vi "Register and Use Kernel Events.vi"() -> ()   [LabVIEW 2012]
uses:
  User Controls/Array Dimensions.ctl
  Non-User VIs/Allocate Memory/AllocateMemory_32f.vi
  Non-User VIs/Set Kernel Arguments/Set Kernel Arguments Memory Object.vi
  Non-User VIs/Error Checking/View Error Log Mode Functional Global.vi
  Non-User VIs/Read Memory/ReadMemory_32f.vi
  OpenCLV x64.lvlib
panel:
  out "Intensity Graph":sgl[][](graph)
  in  "Stop Button":bool
  in  "Slider":dbl(slide) scale=0.0..10.0
  in  "Gauge":dbl(knob) scale=0.0..10.0
  in  "Test Events":bool
  # "Press Test Events and still have control over the UI"
  # "Note:  If running on the CPU, the processer usage will hit 100%, but there is still UI control\nTry running on a GPU as well, though it may finish very quickly!"
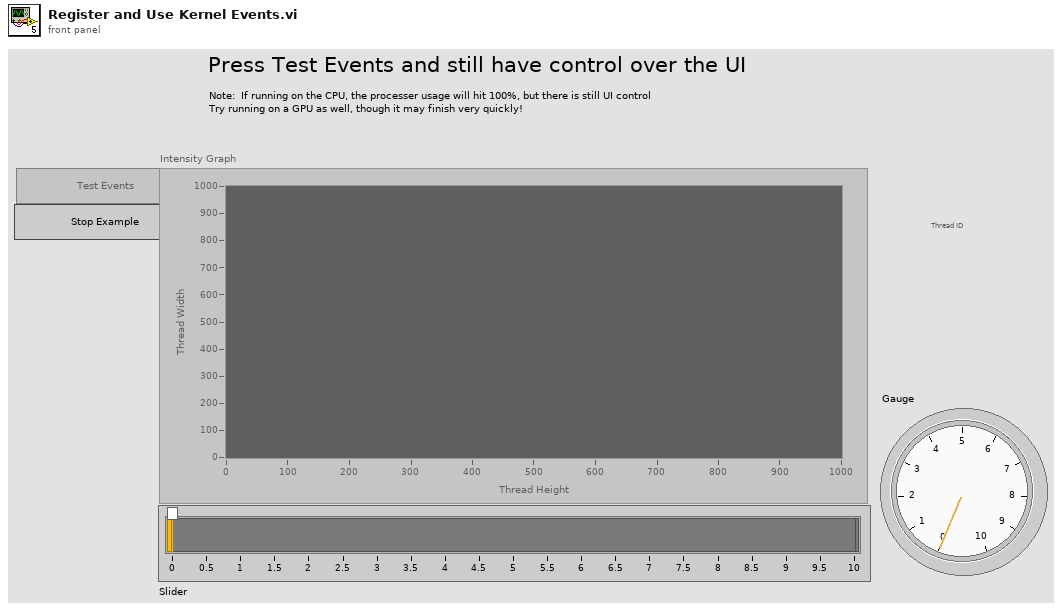
[diagram p1: front panel]
types:
  T1 = enum8{"Enabled", "Disabled", "Disabled and Grayed Out"}
  T2 = typedef "Array Dimensions.ctl" = cluster{"Depth":u64, "Height":u64, "Width":u64}
  T3 = typedef "OpenCLV x64.lvlib/Device ID.ctl" = u64
  T4 = typedef "OpenCLV x64.lvlib/Memory Object.ctl" = cluster{"Device ID":T3, "Memeroy ID":T5, "Dimension":T2, "Memory Type":T6}
  T5 = typedef "OpenCLV x64.lvlib/Memory ID.ctl" = u64
  T6 = typedef "OpenCLV x64.lvlib/Memory Type.ctl" = enum16{"32f", "u8", "i8", "u16", "i16", "u32", "i32", "64f"}
  T7 = typedef "OpenCLV x64.lvlib/Program Handle.ctl" = u64
  T8 = typedef "OpenCLV x64.lvlib/Kernel Handle.ctl" = u64
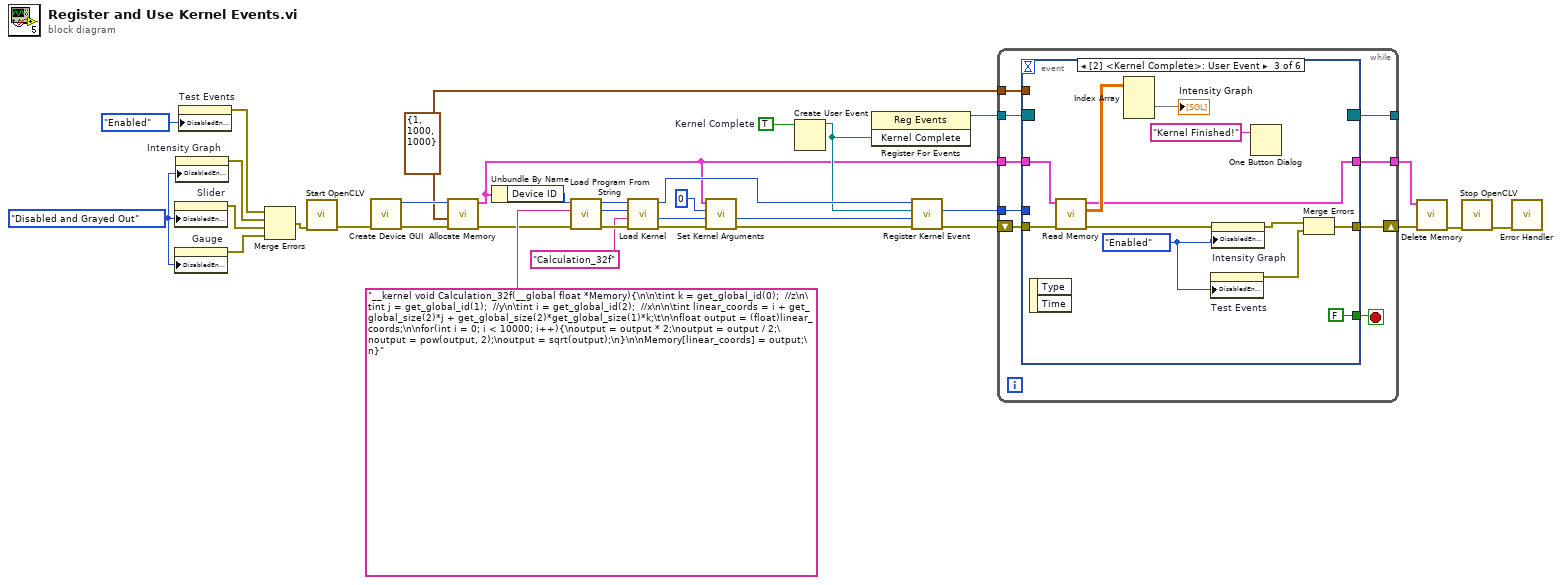
[diagram p0: block diagram]
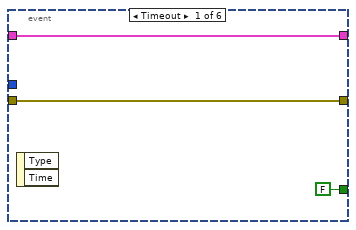
[diagram p2: hidden frame]
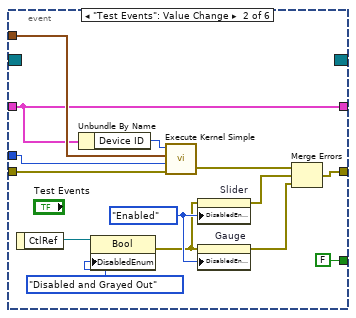
[diagram p3: hidden frame]
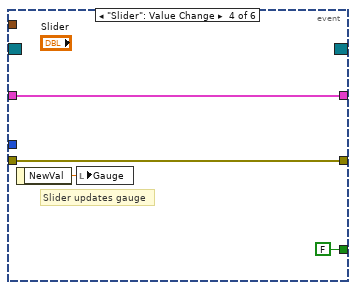
[diagram p4: hidden frame]
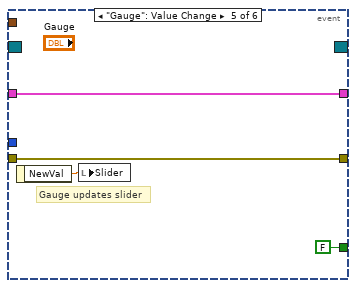
[diagram p5: hidden frame]
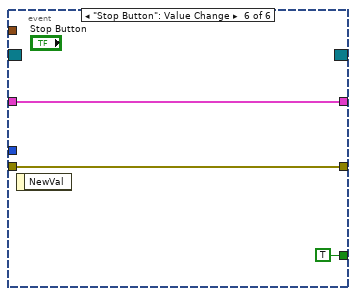
[diagram p6: hidden frame]
diagram:
  w13 = T1."Disabled and Grayed Out" ("Disabled")
  w24 = T2 {"Depth"=1, "Height"=1000, "Width"=1000} ("Dimension")
  w28 = TRUE  # Kernel Complete
  n1 = property on="Slider" class="Slide (strict)"("DisabledEnum"=w13) -> (error out=w17:errorcluster)  [unwired: 2 in, 1 out]
  n2 = property on="Gauge" class="Knob (strict)"("DisabledEnum"=w13) -> (error out=w16:errorcluster)  [unwired: 2 in, 1 out]
  n3 = property on="Intensity Graph" class="IntGraph (strict)"("DisabledEnum"=w13) -> (error out=w12:errorcluster)  [unwired: 2 in, 1 out]
  n4 = property on="Test Events" class="Bool"("DisabledEnum"=T1."Enabled" ("Disabled")) -> (error out=w10:errorcluster)  [unwired: 2 in, 1 out]
  n5 = Merge Errors(w10, w12, w17, w16) -> (w18:errorcluster)
  n6 = call "Start OpenCLV.vi"("Error In"=w18) -> ("Error Out"=w34:errorcluster)  [unwired: 10 in]
  n7 = call "Create Device GUI.vi"("Error In"=w34) -> ("error constant"=w26:errorcluster, "Device Reference"=w25:T3)  [unwired: 9 in]
  n8 = call-poly "Allocate Memory.vi"("Error In"=w26, "Dimension"=w24, "Device In"=w25) -> ("Error Out"=w23:errorcluster, "Memory Object"=w3:T4)  [unwired: 6 in, 1 out]
  n9 = Unbundle By Name(w3) -> ("Device ID"=w19:T3)
  n10 = call "Load Program From String.vi"("Error In"=w23, "OpenCL Source Code"="__kernel void Calculation_32f(__global float *Memory){\n\n\tint k = get_global_id(0);  //z\n\tint j = get_global_id(1);  //y\n\tint i = get_global_id(2);  //x\n\n\tint linear_coords = i + get_global_size(2)*j + get_global_size(2)*get_global_size(1)*k;\t\n\nfloat output = (float)linear_coords;\n\nfor(int i = 0; i < 10000; i++){\noutput = output * 2;\noutput = output / 2;\noutput = pow(output, 2);\noutput = sqrt(output);\n}\n\nMemory[linear_coords] = output;\n}", "Device In"=w19) -> ("Error Out"=w31:errorcluster, "Program Handle"=w30:T7, "Device Out"=w32:T3)  [unwired: 6 in]
  n11 = call "Load Kernel.vi"("Error In"=w31, "Kernel Name"="Calculation_32f", "Program Handle"=w30, "Device In"=w32) -> ("Error Out"=w22:errorcluster, "Kernel Handle"=w21:T8, "Device Out"=w6:T3)  [unwired: 4 in, 1 out]
  n12 = call-poly "Set Kernel Arguments.vi"("Error In"=w22, "Kernel Handle"=w21, "Argument Number"=0, "Memory Object"=w3) -> ("Error Out"=w8:errorcluster, "Kernel Handle out"=w7:T8)  [unwired: 5 in, 1 out]
  n13 = Create User Event(user event datatype=w28) -> (user event=w5:refnum<user-event>)  [unwired: 1 in, 1 out]
  n14 = register-events(w5) -> (reference out=w27:refnum<event-registration>)  [unwired: 2 in, 1 out]
  n15 = call "Register Kernel Event.vi"("Error In"=w8, "Kernel Handle"=w7, "User Event"=w5, "Device ID"=w6) -> ("Error Out"=w9:errorcluster, "Kernel Handle Out"=w1:T8)  [unwired: 4 in, 2 out]
  n16 = while {
    tunnel: w27 -> [w43]
    tunnel: w24 -> [w40]
    shift-right: [w39] -> w14
    shift-left: w9 -> [w42]
    tunnel: [w38] -> _
    tunnel: w3 -> [w37]
    tunnel: [w36] -> w4
    tunnel: w1 -> [w35]
    stop <- w41 stop-if-true
    n17 = event shown="[2] <Kernel Complete>: User Event" {
      selector: w43 -> [_ _ _ _ _ _]
      dyn-events: [_ _ _ _ _ _] -> w38
      timeout: _ -> [_ _ _ _ _ _]
      tunnel: w42 -> [w45 w60 w71 w74 w78 w83]
      tunnel: [FALSE FALSE FALSE FALSE FALSE TRUE] -> w41
      tunnel: w40 -> [_ w59 _ _ _ _]
      tunnel: [w45 w54 w69 w74 w78 w83] -> w39
      tunnel: w37 -> [w44 w48 w62 w73 w77 w81]
      tunnel: [w44 w48 w61 w73 w77 w81] -> w36
      tunnel: w35 -> [_ w47 _ _ _ _]
      event Timeout {
        n18 = event-data() -> ()  [unwired: 1 in, 2 out]
      }
      event "Test Events": Value Change {
        w58 = T1."Enabled" ("Disabled")
        n19 = event-data() -> ("CtlRef"=w57:refnum<vi>)  [unwired: 1 in]
        n20 = Unbundle By Name(w48) -> ("Device ID"=w49:T3)
        n21 = property class="Bool"(reference=w57, "DisabledEnum"=T1."Disabled and Grayed Out" ("Disabled")) -> (error out=w55:errorcluster)  [unwired: 1 in, 1 out]
        n22 = call "Execute Kernel Simple.vi"("Error In"=w60, "Kernel Handle"=w47, "Thread Dimensions"=w59, "Device In"=w49) -> ("Error Out"=w51:errorcluster)  [unwired: 4 in, 3 out]
        n23 = property on="Slider" class="Slide (strict)"(error in=w55, "DisabledEnum"=w58) -> (error out=w52:errorcluster)  [unwired: 1 in, 1 out]
        n24 = property on="Gauge" class="Knob (strict)"(error in=w55, "DisabledEnum"=w58) -> (error out=w53:errorcluster)  [unwired: 1 in, 1 out]
        n25 = Merge Errors(w51, w52, w53) -> (w54:errorcluster)
      }
      event User Event {
        w63 = T1."Enabled" ("Disabled")
        n26 = event-data() -> ()  [unwired: 1 in, 2 out]
        n27 = call-poly "Read Memory.vi"("Error In"=w71, "Memory Object In"=w62) -> ("Error Out"=w65:errorcluster, "Data Out"=w67:sgl[][][], "Memory Object Out"=w61:T4)  [unwired: 6 in, 1 out]
        n28 = Index Array(array=w67) -> (element=→"Intensity Graph":sgl[][])  [unwired: 3 in]
        n29 = property on="Test Events" class="Bool"("DisabledEnum"=w63) -> (error out=w68:errorcluster)  [unwired: 2 in, 1 out]
        n30 = property on="Intensity Graph" class="IntGraph (strict)"(error in=w65, "DisabledEnum"=w63) -> (error out=w64:errorcluster)  [unwired: 1 in, 1 out]
        n31 = One Button Dialog(message="Kernel Finished!") -> ()  [unwired: 1 in, 1 out]
        n32 = Merge Errors(w64, w68) -> (w69:errorcluster)
      }
      event "Slider": Value Change {
        # "Slider updates gauge"
        n33 = event-data() -> ("NewVal"=w76:dbl)  [unwired: 1 in]
        n34 = local write "Gauge"(w76) -> ()
      }
      event "Gauge": Value Change {
        # "Gauge updates slider"
        n35 = event-data() -> ("NewVal"=w80:dbl)  [unwired: 1 in]
        n36 = local write "Slider"(w80) -> ()
      }
      event "Stop Button": Value Change {
        n37 = event-data() -> ()  [unwired: 1 in, 1 out]
      }
    }
  }
  n38 = call "Delete Memory.vi"("Error In"=w14, "Memory Object In"=w4) -> ("Error Out"=w15:errorcluster)  [unwired: 8 in, 1 out]
  n39 = call "Stop OpenCLV.vi"("Error In"=w15) -> ("Error Out"=w2:errorcluster)  [unwired: 10 in]
  n40 = call-poly "Error Handler.vi"("Error In"=w2) -> ()  [unwired: 10 in, 1 out]
